vi "[Bug] Double FFT Mesurament RT with Frequency Linearization & BackNoise Remove Test.vi"() -> ()   [LabVIEW 2014]
uses:
  <vilib>/Platform/TimedLoop/XDataNode/timing_clust.ctl
  <vilib>/Platform/TimedLoop/XDataNode/nitl_modes.ctl
  <vilib>/Platform/TimedLoop/XDataNode/wakeup.ctl
  <vilib>/FPGAPlugInAG/sbRIO-9636/niLvFpga_Open_sbRIO-9636.vi
  <vilib>/rvi/interface/common/dynamic/niFpgaDynamicAddResources.vi
  <vilib>/FPGAPlugInAG/Dynamic/niLvFpga_Reset_Dynamic.vi
  <vilib>/Utility/error.llb/Error Cluster From Error Code.vi
  <vilib>/rvi/errors/niLvFpgaAdjustHostInterfaceError.vi
  <vilib>/rvi/interface/common/niFpgaWaitOnOcc.vi
  <vilib>/FPGAPlugInAG/Dynamic/niLvFpga_Run_Dynamic.vi
  <vilib>/FPGAPlugInAG/Dynamic/niLvFpga_Abort_Dynamic.vi
  <vilib>/FPGAPlugInAG/Dynamic/niLvFpga_Close_Dynamic.vi
  <vilib>/rvi/interface/nirviOpenFPGA/nirviOpenFPGA.xnode
  FPGA Bitfiles/LaserDistanceSen_FPGATarget_DoubleFFTMesuram_6dDziXQAIGE.lvbitx
  FPGA Target/Test VIs/Double FFT Mesurament Test with Background Noise Remove.vi
  <vilib>/rvi/interface/nirviMethod/nirviMethod.xnode
  <vilib>/rvi/interface/nirviReadWriteControl/nirviReadWriteControl.xnode
  <vilib>/Platform/TimedLoop/XDataNode/XDataNode.xnode
  <vilib>/rvi/interface/nirviCloseFPGA/nirviCloseFPGA.xnode
  <vilib>/FPGAPlugInAG/Dynamic/niLvFpga_ConfigureFifo_Dynamic.vi
  <vilib>/rvi/errors/niLvFpgaMergeErrorWithErrorCode.vi
  <vilib>/FPGAPlugInAG/Dynamic/niLvFpga_StartFifo_Dynamic.vi
  <vilib>/rvi/interface/Simulation/niFpgaSimulationCallBeginRW.vi
  <vilib>/FPGAPlugInAG/Dynamic/niLvFpga_ReadFifo_Dynamic.vi
  <vilib>/Platform/TimedLoop/XDataNode/XDNodeRunTimeDep.lvlib
  NiFpgaLv.dll
panel:
  in  "polynomial order":i32=3
  in  "side points":i32=6
  out "2^(n-bit) misure mediate":dbl
  in  "n-bit":i32=10
  in  "SubtractionType":T1(ring)
  out "Fondo Signal":dbl[](graph)
  in  "LowPass Filter: Low cutoff frequency":dbl=20000.0 format="%#_13g"
  in  "PolyFitting: Poly Grade":dbl=12.0
  in  "Scale Factor Rising":dbl=0.5
  out "2) Std Dev":dbl
  out "1) Std Dev":dbl
  in  "Scale Factor Falling":dbl=0.5
  in  "Triangolo dritto":bool=TRUE
  in  "Acrive  Smooth":bool
  out "Complete SkewTri":dbl[](graph)
  out "2) Tri edge RISING":dbl[](graph)
  out "1) Tri edge FALLING":dbl[](graph)
  out "1) Ext Mean Time Curve":dbl[](graph)
  out "2) Ext Mean Time Curve":dbl[](graph)
  out "2) Mean Freq Curve Rising":dbl[](graph)
  out "1) Mean Freq Curve Falling":dbl[](graph)
  out "2) Freq curve":dbl[](graph)
  out "1) Freq curve":dbl[](graph)
  in  "FFT Sliding Win Size":i32=128
  out "1) SmoothSubSig":dbl[](graph)
  out "2) SmoothSubSig":dbl[](graph)
  in  "Acrive Fit":bool=TRUE
  in  "Poly Order":i32=3
  in  "Side points":i32=13
  in  "Poly Grade":dbl=5.0
  out "2) Signal&Fit 2":dbl[][](graph)
  out "1) Signal&Fit":dbl[][](graph)
  in  "tieni premuto per":i32=1
  out "Current Sig lin":i32
  in  "Acrive Linearization":bool
  in  "# Measurements for Linearization":i32=10
  in  "?":bool
  out "maxbin_secondFFT":i32
  out "maxbin_firstFFT":i32
  out "f_rise":dbl
  out "f_fall":dbl
  out "f_mean":dbl
  out "Velocity (m/s)":dbl
  out "Distance (m)":dbl
  in  "Initial Latency points":u32(slide) scale=0.0..1249.0
  out "Second FFT (bin)":dbl[](graph)
  out "Second Signal (points) - Rising Triangular":dbl[](graph)
  out "First FFT (bin)":dbl[](graph)
  out "First Signal (points) - Falling Triangular":dbl[](graph)
  in  "Snapshot":bool
  in  "Windowing":T2(ring)
  in  "first bin":i32=5
  in  "last bin":i32=255
  in  "lower limit 2":u32(slide)=738 scale=625.0..738.0
  in  "lower limit 1":u32(slide)=113 scale=0.0..113.0
  # "-> TODO: Sistemare problema della finestra di acquisizione ritardata"
  # "Estrazione del rumore di fondo (Background noise extraction)"
  # "Sav Golay Filter"
  # "WARNING:\nOnce pressed wait untill the end of operation"
  # "OFFLINE parameters"
  # "Triangolo storto\nda costante"
  # "Max Detection FFT bin range"
  # "ONLINE parameters"
  # "Se la sottrazione del fondo non è eseguita su FPGA.\n Attivarla per eseguirla lato RT"
  # "Smoothing (S-G Params)"
  # "Fitting"
  # "ONLY POWER OF 2"
  # "Min: 2 Max: 256 (2, 4, 8, 16, 32, 64, 128, 256)"
  # "LINEARIZATION FINAL RESULTS"
  # "dev standard (max-min)"
  # "%"
  # "%"
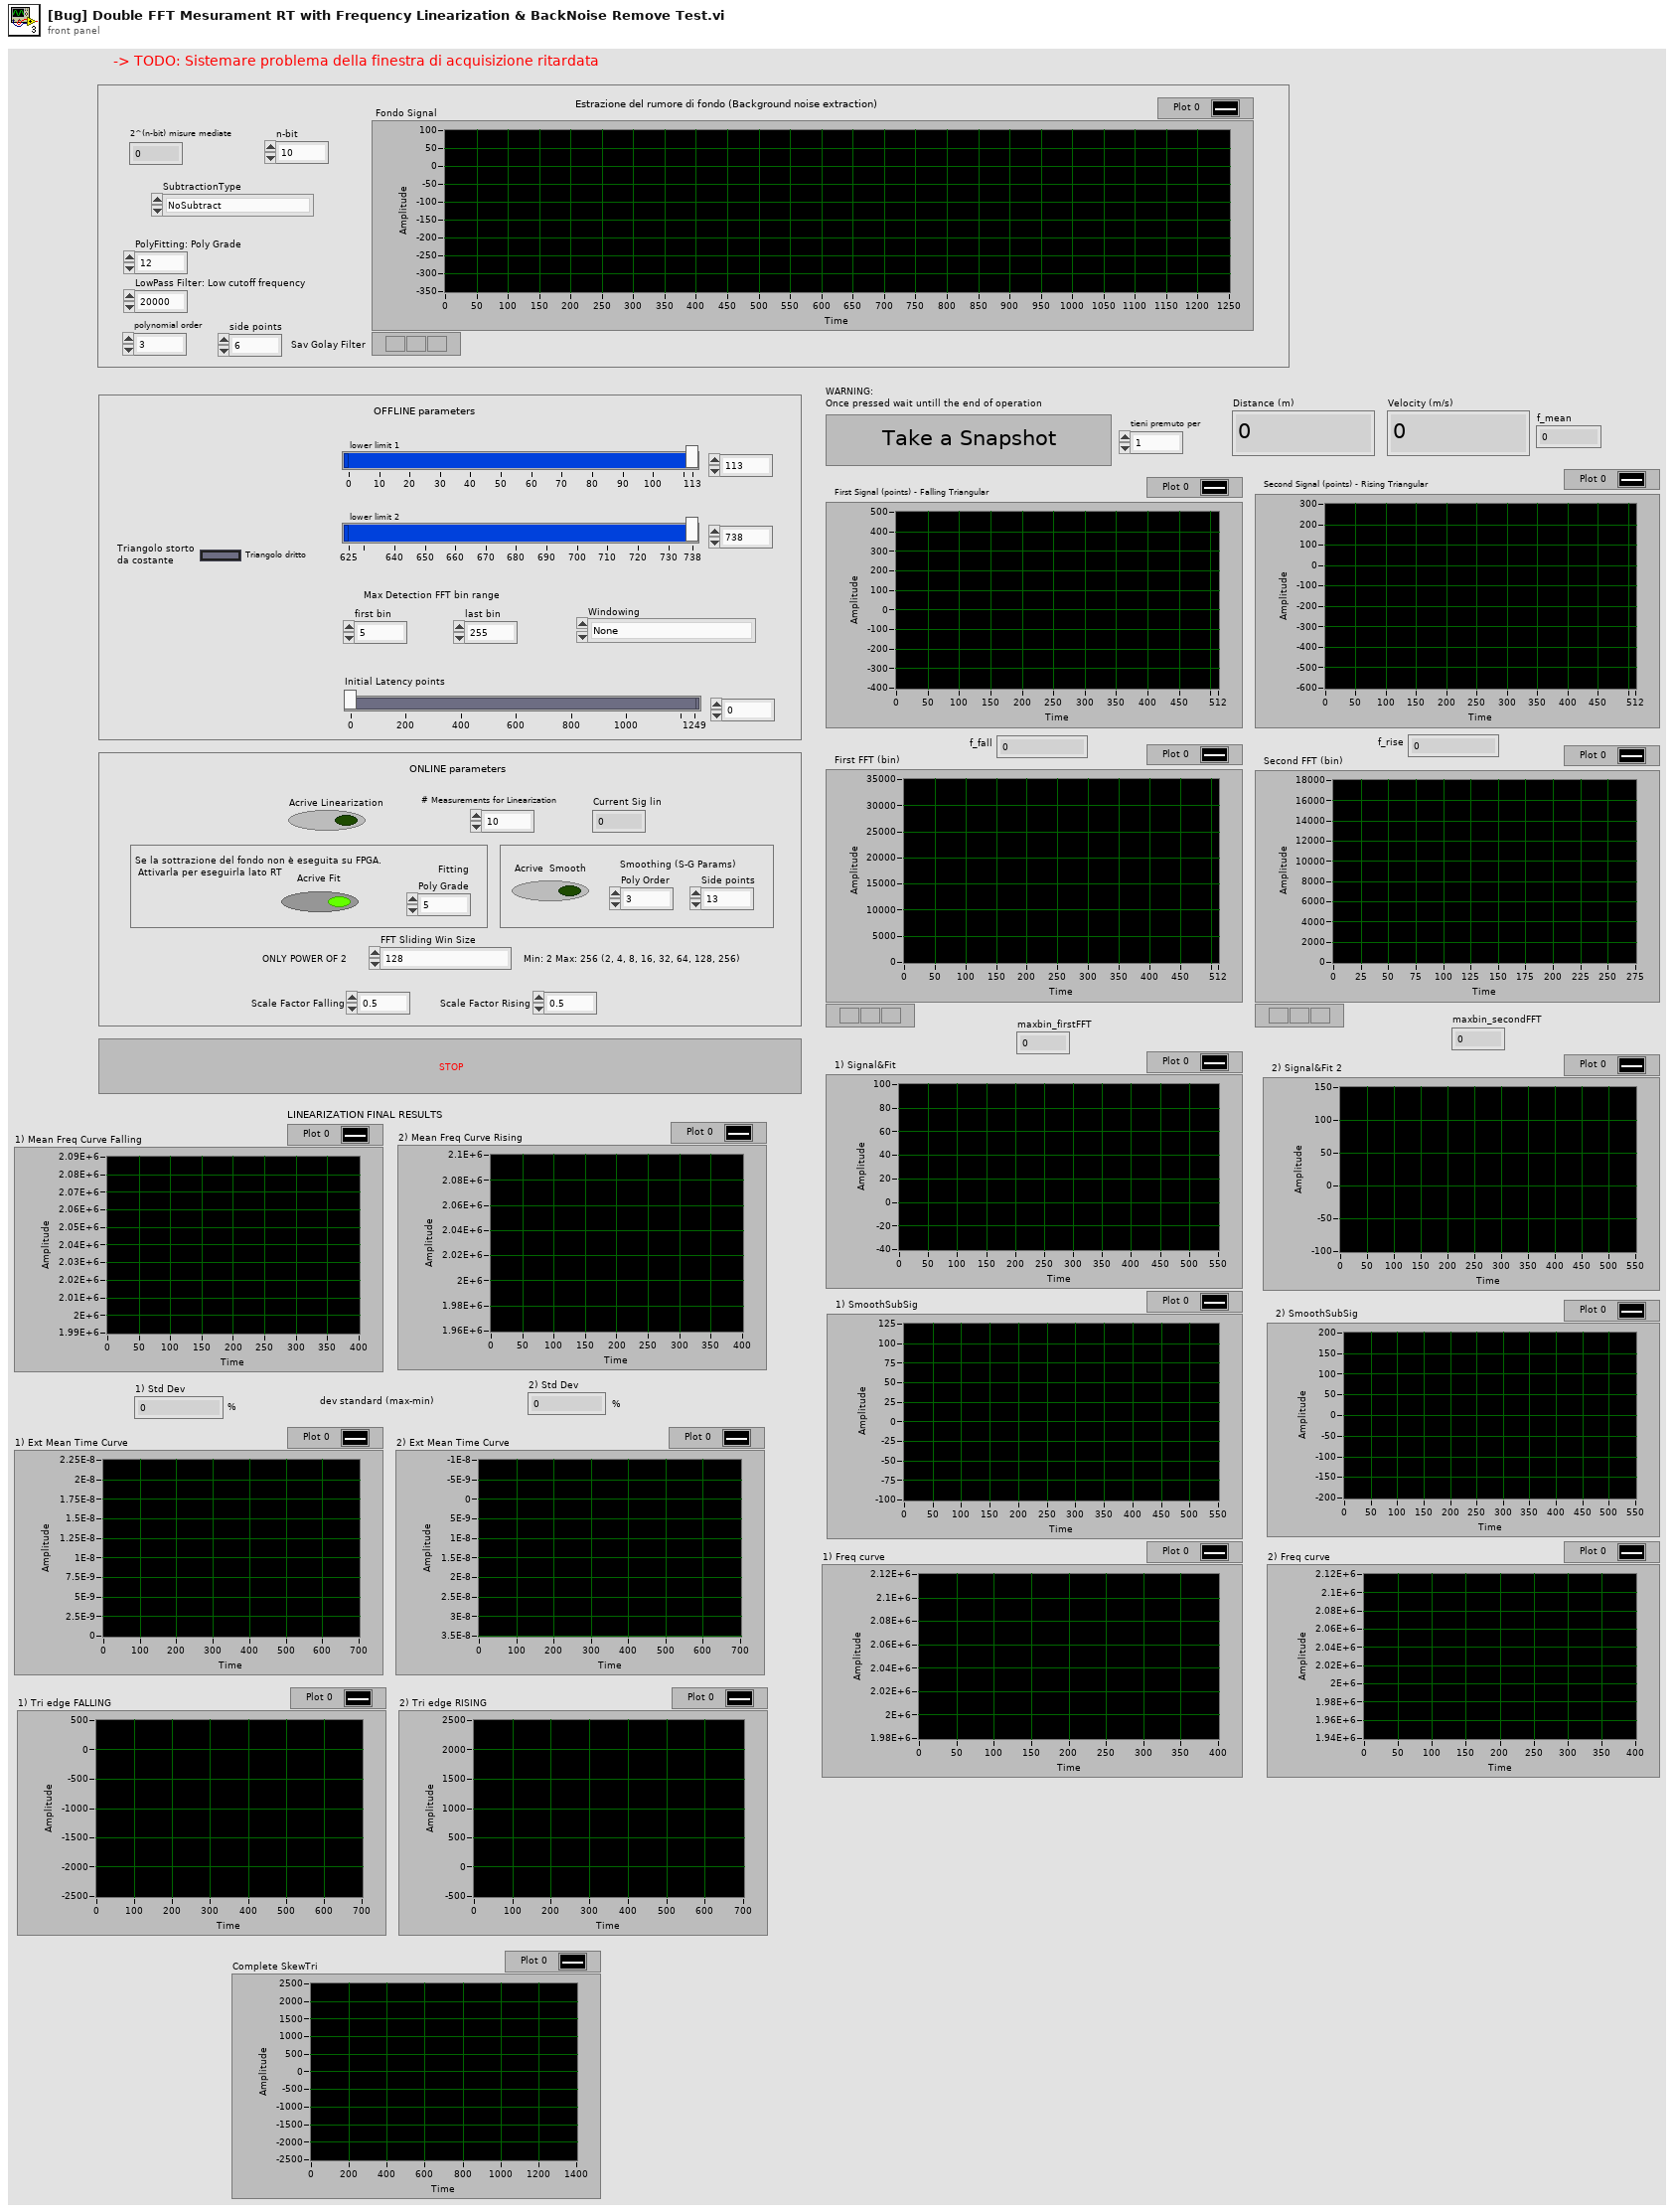
[diagram p1: front panel]
types:
  T1 = enum16{"NoSubtract", "StartingCurve", "LowPass", "PolyFitting", "SavGolay"}
  T2 = enum16{"None", "Hanning", "Hamming", "Blackman", "Blackman-Harris"}
  T3 = typedef "XDNodeRunTimeDep.lvlib/timing_clust.ctl" = cluster{"Expected End [f-1]":u64, "Actual End [f-1]":u64, "Finished Late? [f-1]":bool, "Expected End [i-1]":u64, "Actual End [i-1]":u64, "Finished Late? [i-1]":bool, "Expected Start [i]":u64, "Actual Start [i]":u64, "Expected Start [f]":u64, "Actual Start [f]":u64, "Source Name":string, "Structure Name":string, "Period":i64, "Deadline":i64, "Offset":i64, "Start":i64, "Priority":i32, "Timeout":i32, "Mode":T4, "Wakeup Reason":T5, "Error":errorcluster, "Source Type":string, "Secondary Source Type":string, "Global End Time":u64, "Global Start Time":u64, "Frame Duration":u64, "Iteration Duration":u64, "Assigned CPU":i32, "I/O Scan Engine Mode":u32}
  T4 = typedef "XDNodeRunTimeDep.lvlib/nitl_modes.ctl" = enum32{"No Change", "Process missed periods, maintain original phase", "Discard missed periods, maintain original phase", "Process missed periods, ignore original phase", "Discard missed periods, ignore original phase"}
  T5 = typedef "XDNodeRunTimeDep.lvlib/wakeup.ctl" = enum32{"Normal", "Aborted", "Asynchronous wakeup", "Timing source error", "Timed loop error", "Timeout"}
  T6 = typedef "NI_Matrix.lvlib/RealMatrix.ctl" = dbl[][]
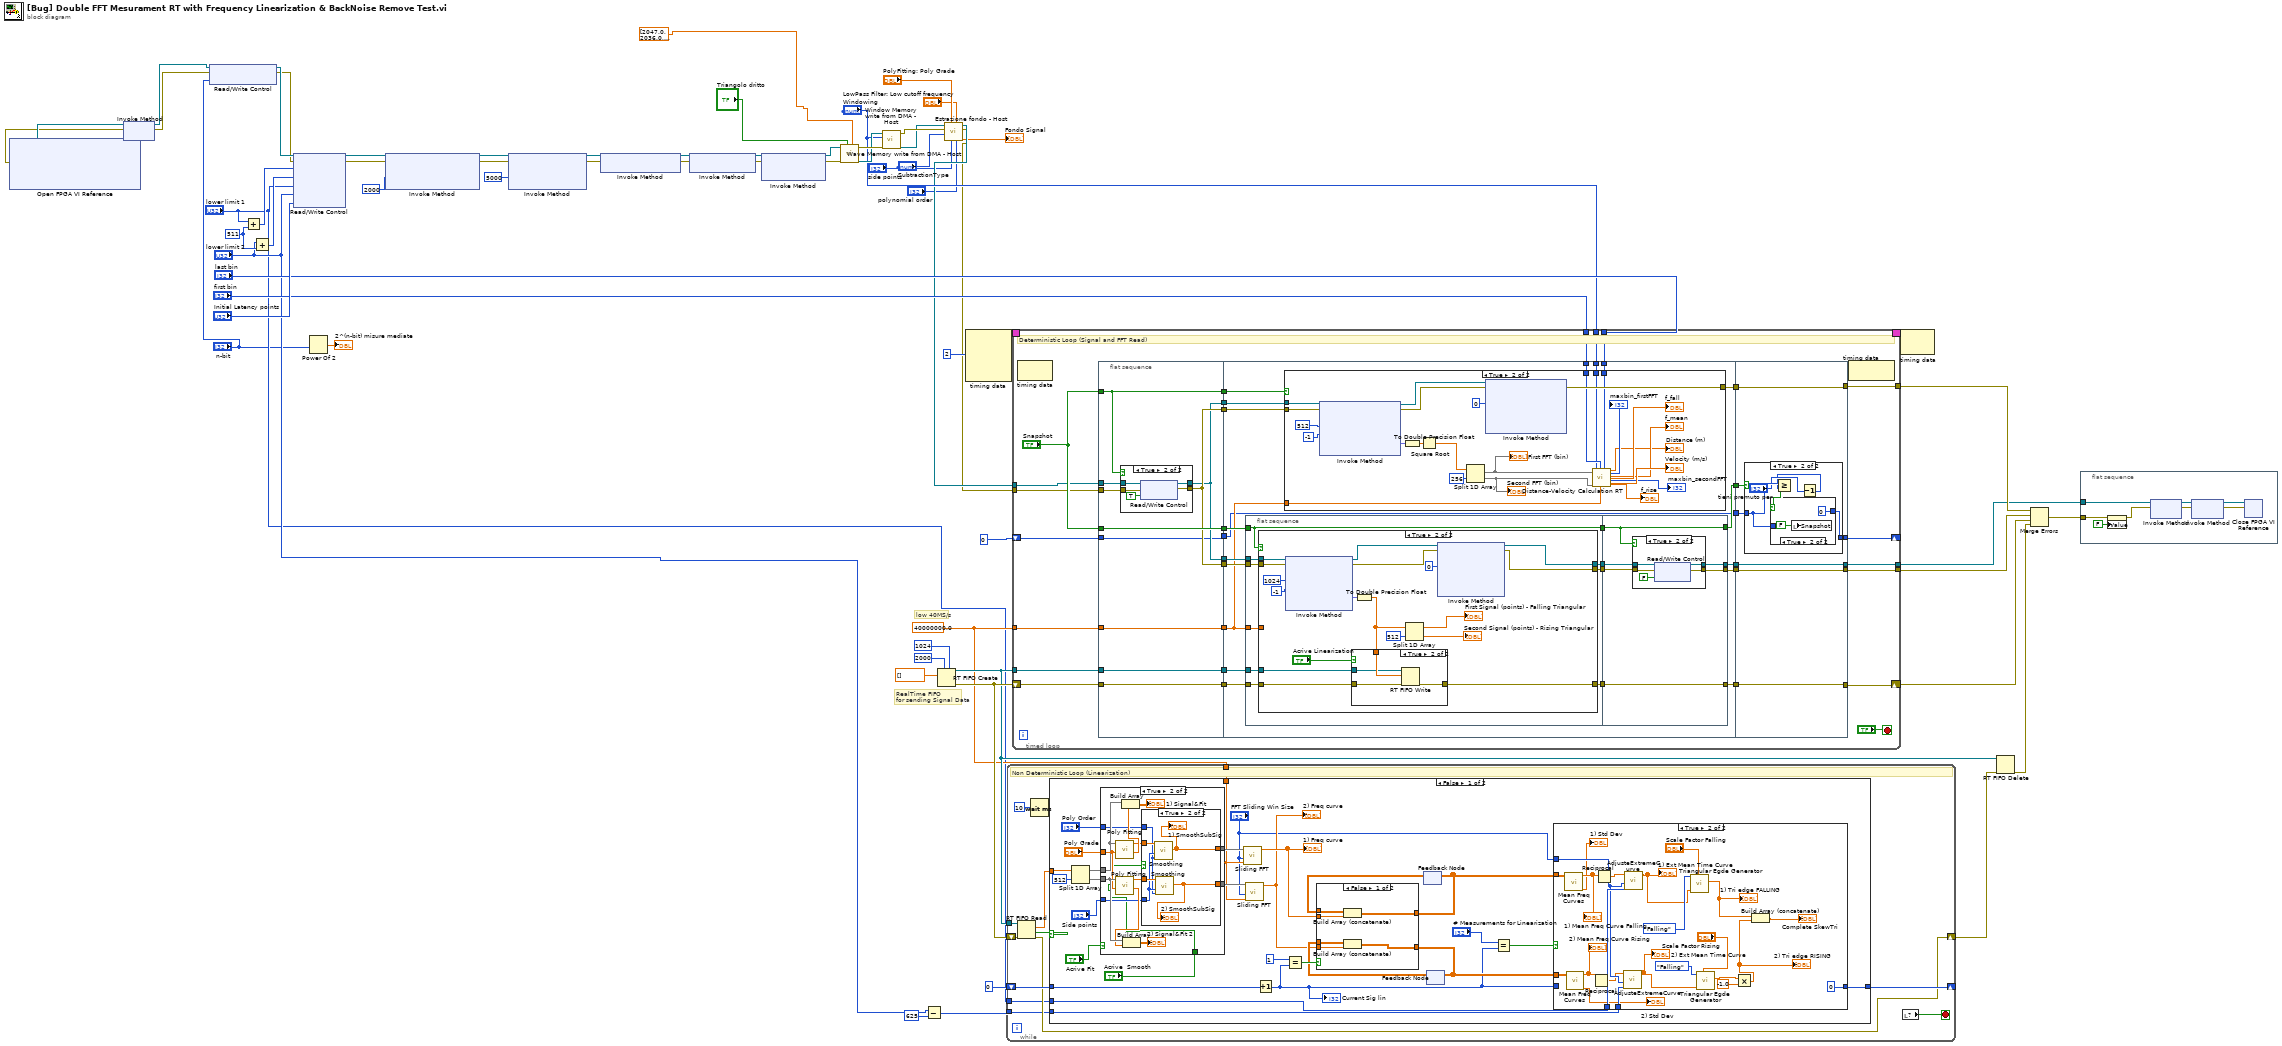
[diagram p0: block diagram]
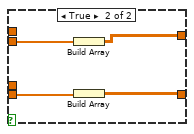
[diagram p5: hidden frame]
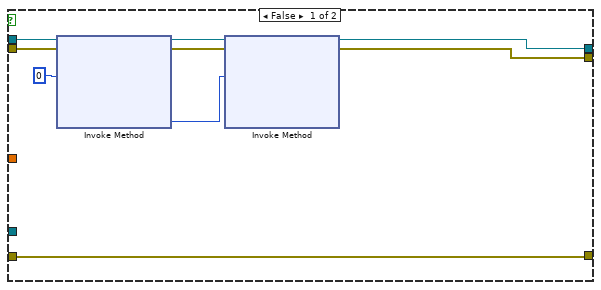
[diagram p8: hidden frame]
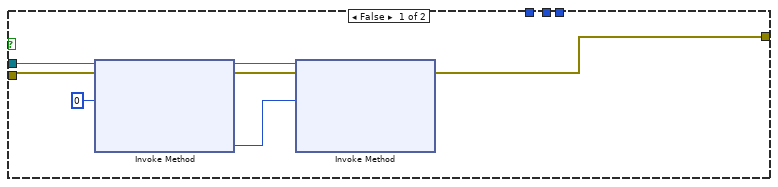
[diagram p11: hidden frame]
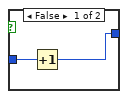
[diagram p13: hidden frame]
diagram:
  w63 = u32 511 ("y")
  w22 = 40000000.0 ("Sample Rate (S/s)")
  # "RealTime FIFO \nfor sending Signal Data"
  # "low 40MS/s"
  n1 = xnode "Open FPGA VI Reference"() -> ("FPGA VI Reference Out"=w7:refnum<k20>, "error out"=w6:errorcluster)  [unwired: 2 in]
  n2 = xnode "Invoke Method"("FPGA VI Reference In"=w7, "error in"=w6) -> ("FPGA VI Reference Out"=w4:refnum<k20>, "error out"=w2:errorcluster)
  n3 = xnode "Read/Write Control"("FPGA VI Reference In"=w4, "error in"=w2, "n-bit (2^nbit medie)"="n-bit") -> ("FPGA VI Reference Out"=w3:refnum<k20>, "error out"=w1:errorcluster)
  n4 = Add(x="lower limit 1", y=w63) -> (x+y=w65:u32)
  n5 = Add(x="lower limit 2", y=w63) -> (x+y=w64:u32)
  n6 = xnode "Read/Write Control"("FPGA VI Reference In"=w3, "error in"=w1, "upper limit 1"=w65, "upper limit 2"=w64, "lower limit 1"="lower limit 1", "lower limit 2"="lower limit 2", "Latency points"="Initial Latency points") -> ("FPGA VI Reference Out"=w62:refnum<k20>, "error out"=w61:errorcluster)
  n7 = Power Of 2(x="n-bit") -> (2^x=→"2^(n-bit) misure mediate":dbl)
  n8 = xnode "Invoke Method"("FPGA VI Reference In"=w62, "error in"=w61, "Requested Depth"=u32 2000) -> ("FPGA VI Reference Out"=w40:refnum<k20>, "error out"=w41:errorcluster)  [unwired: 1 out]
  n9 = xnode "Invoke Method"("FPGA VI Reference In"=w40, "error in"=w41, "Requested Depth"=u32 5000) -> ("FPGA VI Reference Out"=w54:refnum<k20>, "error out"=w55:errorcluster)  [unwired: 1 out]
  n10 = xnode "Invoke Method"("FPGA VI Reference In"=w54, "error in"=w55) -> ("FPGA VI Reference Out"=w38:refnum<k20>, "error out"=w39:errorcluster)
  n11 = xnode "Invoke Method"("FPGA VI Reference In"=w38, "error in"=w39) -> ("FPGA VI Reference Out"=w52:refnum<k20>, "error out"=w53:errorcluster)
  n12 = xnode "Invoke Method"("FPGA VI Reference In"=w52, "error in"=w53) -> ("FPGA VI Reference Out"=w58:refnum<k20>, "error out"=w57:errorcluster)  [unwired: 1 in]
  n13 = call "Wave Memory write from DMA - Host.vi"("Custom Triangular Signal (fal-ris)"=dbl[] [2047.0, 2036.0, 2024.0, 2013.0, 2002.0, 1990.0, 1979.0, 1968.0, 1956.0, 1945.0, 1934.0, 1923.0, 1912.0, 1900.0, 1889.0, 1878.0, 1867.0, 1856.0, 1845.0, 1833.0, 1822.0, 1811.0, 1800.0, 1789.0, 1778.0, 1767.0, 1756.0, 1745.0, 1734.0, 1723.0, 1712.0, 1702.0, 1691.0, 1680.0, 1669.0, 1658.0, 1647.0, 1636.0, 1626.0, 1615.0, 1604.0, 1593.0, 1583.0, 1572.0, 1561.0, 1550.0, 1540.0, 1529.0, 1518.0, 1508.0, 1497.0, 1487.0, 1476.0, 1465.0, 1455.0, 1444.0, 1434.0, 1423.0, 1413.0, 1402.0, 1392.0, 1381.0, 1371.0, 1360.0, 1350.0, 1340.0, 1329.0, 1319.0, 1309.0, 1298.0, 1288.0, 1278.0, 1267.0, 1257.0, 1247.0, 1237.0, 1226.0, 1216.0, 1206.0, 1196.0, 1186.0, 1176.0, 1165.0, 1155.0, 1145.0, 1135.0, 1125.0, 1115.0, 1105.0, 1095.0, 1085.0, 1075.0, 1065.0, 1055.0, 1045.0, 1035.0, 1025.0, 1015.0, 1006.0, 996.0, 986.0, 976.0, 966.0, 956.0, 947.0, 937.0, 927.0, 917.0, 908.0, 898.0, 888.0, 879.0, 869.0, 859.0, 850.0, 837.0, 826.0, 816.0, 804.0, 796.0, 788.0, 778.0, 769.0, 758.0, 750.0, 743.0, 733.0, 724.0, 717.0, 709.0, 701.0, 693.0, 686.0, 677.0, 669.0, 661.0, 653.0, 645.0, 638.0, 630.0, 622.0, 615.0, 607.0, 599.0, 592.0, 583.0, 576.0, 569.0, 561.0, 554.0, 547.0, 539.0, 532.0, 525.0, 518.0, 509.0, 501.0, 492.0, 486.0, 478.0, 471.0, 463.0, 456.0, 450.0, 442.0, 435.0, 429.0, 421.0, 415.0, 408.0, 401.0, 394.0, 388.0, 381.0, 375.0, 368.0, 361.0, 355.0, 349.0, 342.0, 336.0, 330.0, 323.0, 317.0, 311.0, 304.0, 298.0, 292.0, 286.0, 279.0, 273.0, 267.0, 261.0, 255.0, 249.0, 242.0, 236.0, 230.0, 224.0, 218.0, 212.0, 206.0, 200.0, 194.0, 187.0, 181.0, 175.0, 169.0, 163.0, 157.0, 150.0, 144.0, 138.0, 132.0, 125.0, 119.0, 113.0, 107.0, 101.0, 95.0, 88.0, 82.0, 77.0, 71.0, 65.0, 59.0, 53.0, 47.0, 41.0, 35.0, 29.0, 23.0, 18.0, 11.0, 6.0, 0.0, -6.0, -12.0, -18.0, -23.0, -29.0, -35.0, -41.0, -47.0, -52.0, -58.0, -64.0, -69.0, -75.0, -81.0, -87.0, -92.0, -98.0, -104.0, -109.0, -115.0, -121.0, -126.0, -132.0, -138.0, -144.0, -149.0, -155.0, -161.0, -166.0, -172.0, -177.0, -183.0, -189.0, -194.0, -200.0, -205.0, -211.0, -216.0, -222.0, -227.0, -233.0, -238.0, -244.0, -249.0, -255.0, -260.0, -266.0, -271.0, -277.0, -283.0, -288.0, -294.0, -299.0, -304.0, -310.0, -315.0, -321.0, -326.0, -331.0, -337.0, -342.0, -348.0, -353.0, -358.0, -364.0, -369.0, -375.0, -380.0, -385.0, -391.0, -396.0, -402.0, -407.0, -413.0, -418.0, -423.0, -429.0, -434.0, -439.0, -445.0, -450.0, -456.0, -461.0, -466.0, -472.0, -477.0, -483.0, -488.0, -493.0, -499.0, -504.0, -510.0, -515.0, -520.0, -526.0, -531.0, -537.0, -542.0, -548.0, -553.0, -558.0, -564.0, -569.0, -574.0, -580.0, -585.0, -590.0, -596.0, -601.0, -606.0, -612.0, -617.0, -622.0, -628.0, -633.0, -638.0, -644.0, -649.0, -654.0, -660.0, -665.0, -670.0, -676.0, -681.0, -686.0, -692.0, -697.0, -702.0, -708.0, -713.0, -718.0, -723.0, -729.0, -734.0, -739.0, -744.0, -750.0, -755.0, -760.0, -765.0, -771.0, -776.0, -781.0, -786.0, -792.0, -797.0, -802.0, -807.0, -812.0, -818.0, -823.0, -828.0, -833.0, -839.0, -844.0, -849.0, -854.0, -859.0, -865.0, -870.0, -875.0, -880.0, -885.0, -891.0, -896.0, -901.0, -906.0, -911.0, -916.0, -922.0, -927.0, -932.0, -937.0, -943.0, -948.0, -953.0, -958.0, -963.0, -969.0, -974.0, -979.0, -984.0, -989.0, -995.0, -1000.0, -1005.0, -1010.0, -1015.0, -1021.0, -1026.0, -1031.0, -1036.0, -1041.0, -1047.0, -1052.0, -1057.0, -1062.0, -1067.0, -1073.0, -1078.0, -1083.0, -1088.0, -1093.0, -1099.0, -1104.0, -1109.0, -1114.0, -1119.0, -1124.0, -1130.0, -1135.0, -1140.0, -1145.0, -1150.0, -1156.0, -1161.0, -1166.0, -1171.0, -1176.0, -1182.0, -1187.0, -1192.0, -1197.0, -1202.0, -1207.0, -1213.0, -1218.0, -1223.0, -1228.0, -1233.0, -1238.0, -1244.0, -1249.0, -1254.0, -1259.0, -1264.0, -1269.0, -1275.0, -1280.0, -1285.0, -1290.0, -1295.0, -1300.0, -1305.0, -1311.0, -1316.0, -1321.0, -1326.0, -1331.0, -1336.0, -1342.0, -1347.0, -1352.0, -1357.0, -1362.0, -1367.0, -1372.0, -1378.0, -1383.0, -1388.0, -1393.0, -1398.0, -1403.0, -1408.0, -1414.0, -1419.0, -1424.0, -1429.0, -1434.0, -1439.0, -1444.0, -1450.0, -1455.0, -1460.0, -1465.0, -1470.0, -1475.0, -1480.0, -1486.0, -1491.0, -1496.0, -1501.0, -1506.0, -1511.0, -1516.0, -1522.0, -1527.0, -1532.0, -1537.0, -1542.0, -1547.0, -1552.0, -1558.0, -1563.0, -1568.0, -1573.0, -1578.0, -1583.0, -1588.0, -1593.0, -1599.0, -1604.0, -1609.0, -1614.0, -1619.0, -1624.0, -1629.0, -1634.0, -1640.0, -1645.0, -1650.0, -1655.0, -1660.0, -1665.0, -1670.0, -1675.0, -1681.0, -1686.0, -1691.0, -1696.0, -1701.0, -1706.0, -1711.0, -1716.0, -1722.0, -1727.0, -1732.0, -1737.0, -1742.0, -1747.0, -1752.0, -1757.0, -1762.0, -1768.0, -1773.0, -1778.0, -1783.0, -1788.0, -1793.0, -1798.0, -1803.0, -1808.0, -1814.0, -1819.0, -1824.0, -1829.0, -1834.0, -1839.0, -1844.0, -1849.0, -1854.0, -1859.0, -1865.0, -1870.0, -1875.0, -1880.0, -1885.0, -1890.0, -1895.0, -1900.0, -1905.0, -1911.0, -1916.0, -1921.0, -1926.0, -1931.0, -1936.0, -1941.0, -1946.0, -1951.0, -1956.0, -1961.0, -1967.0, -1972.0, -1977.0, -1982.0, -1987.0, -1992.0, -1997.0, -2002.0, -2007.0, -2012.0, -2017.0, -2023.0, -2028.0, -2033.0, -2038.0, -2043.0, -2048.0, -2047.0, -2034.0, -2021.0, -2009.0, -1996.0, -1983.0, -1970.0, -1957.0, -1945.0, -1932.0, -1919.0, -1907.0, -1894.0, -1881.0, -1869.0, -1856.0, -1844.0, -1831.0, -1819.0, -1806.0, -1794.0, -1781.0, -1769.0, -1757.0, -1744.0, -1732.0, -1719.0, -1707.0, -1695.0, -1682.0, -1670.0, -1658.0, -1646.0, -1634.0, -1621.0, -1609.0, -1597.0, -1585.0, -1573.0, -1561.0, -1549.0, -1537.0, -1525.0, -1513.0, -1501.0, -1489.0, -1477.0, -1465.0, -1453.0, -1441.0, -1429.0, -1417.0, -1405.0, -1394.0, -1382.0, -1370.0, -1358.0, -1347.0, -1335.0, -1323.0, -1312.0, -1300.0, -1288.0, -1277.0, -1265.0, -1254.0, -1242.0, -1231.0, -1219.0, -1208.0, -1196.0, -1185.0, -1173.0, -1162.0, -1150.0, -1139.0, -1128.0, -1116.0, -1105.0, -1094.0, -1083.0, -1071.0, -1060.0, -1049.0, -1038.0, -1027.0, -1015.0, -1004.0, -993.0, -982.0, -971.0, -960.0, -949.0, -938.0, -927.0, -916.0, -905.0, -894.0, -883.0, -873.0, -862.0, -851.0, -840.0, -829.0, -819.0, -808.0, -797.0, -786.0, -776.0, -765.0, -754.0, -744.0, -733.0, -722.0, -712.0, -697.0, -685.0, -674.0, -661.0, -652.0, -643.0, -632.0, -622.0, -610.0, -602.0, -594.0, -583.0, -574.0, -566.0, -558.0, -550.0, -542.0, -534.0, -525.0, -516.0, -507.0, -499.0, -491.0, -483.0, -475.0, -467.0, -459.0, -451.0, -443.0, -435.0, -426.0, -419.0, -411.0, -404.0, -396.0, -388.0, -381.0, -373.0, -366.0, -359.0, -349.0, -341.0, -331.0, -325.0, -317.0, -309.0, -301.0, -295.0, -288.0, -280.0, -273.0, -266.0, -259.0, -252.0, -246.0, -239.0, -231.0, -225.0, -219.0, -212.0, -205.0, -199.0, -192.0, -186.0, -180.0, -173.0, -167.0, -161.0, -155.0, -148.0, -142.0, -136.0, -130.0, -124.0, -118.0, -112.0, -106.0, -100.0, -94.0, -88.0, -82.0, -76.0, -70.0, -64.0, -58.0, -52.0, -46.0, -40.0, -34.0, -28.0, -21.0, -15.0, -9.0, -3.0, 2.0, 9.0, 15.0, 21.0, 27.0, 33.0, 39.0, 45.0, 51.0, 57.0, 63.0, 69.0, 75.0, 81.0, 86.0, 92.0, 98.0, 103.0, 110.0, 116.0, 121.0, 127.0, 133.0, 138.0, 144.0, 149.0, 155.0, 161.0, 166.0, 172.0, 177.0, 183.0, 189.0, 194.0, 200.0, 205.0, 211.0, 216.0, 221.0, 227.0, 232.0, 238.0, 243.0, 249.0, 254.0, 259.0, 265.0, 270.0, 276.0, 281.0, 286.0, 292.0, 297.0, 303.0, 308.0, 314.0, 319.0, 324.0, 329.0, 335.0, 340.0, 345.0, 351.0, 356.0, 361.0, 366.0, 371.0, 377.0, 382.0, 387.0, 392.0, 397.0, 403.0, 408.0, 413.0, 418.0, 423.0, 429.0, 434.0, 439.0, 444.0, 449.0, 454.0, 459.0, 464.0, 469.0, 474.0, 479.0, 484.0, 489.0, 494.0, 499.0, 504.0, 509.0, 514.0, 520.0, 525.0, 530.0, 535.0, 540.0, 545.0, 550.0, 555.0, 560.0, 565.0, 570.0, 575.0, 580.0, 585.0, 590.0, 595.0, 600.0, 605.0, 610.0, 615.0, 620.0, 625.0, 630.0, 636.0, 641.0, 646.0, 651.0, 656.0, 661.0, 666.0, 671.0, 676.0, 681.0, 686.0, 691.0, 696.0, 701.0, 706.0, 711.0, 716.0, 721.0, 726.0, 731.0, 736.0, 741.0, 746.0, 751.0, 756.0, 761.0, 765.0, 770.0, 775.0, 780.0, 785.0, 790.0, 795.0, 800.0, 805.0, 810.0, 815.0, 820.0, 825.0, 829.0, 834.0, 839.0, 844.0, 849.0, 854.0, 859.0, 864.0, 868.0, 873.0, 878.0, 883.0, 888.0, 893.0, 897.0, 902.0, 907.0, 912.0, 917.0, 921.0, 926.0, 931.0, 936.0, 941.0, 945.0, 950.0, 955.0, 960.0, 965.0, 969.0, 974.0, 979.0, 984.0, 988.0, 993.0, 998.0, 1003.0, 1007.0, 1012.0, 1017.0, 1022.0, 1027.0, 1031.0, 1036.0, 1041.0, 1046.0, 1051.0, 1055.0, 1060.0, 1065.0, 1070.0, 1075.0, 1079.0, 1084.0, 1089.0, 1094.0, 1098.0, 1103.0, 1108.0, 1113.0, 1118.0, 1122.0, 1127.0, 1132.0, 1137.0, 1141.0, 1146.0, 1151.0, 1156.0, 1161.0, 1165.0, 1170.0, 1175.0, 1180.0, 1184.0, 1189.0, 1194.0, 1199.0, 1204.0, 1208.0, 1213.0, 1218.0, 1223.0, 1227.0, 1232.0, 1237.0, 1242.0, 1246.0, 1251.0, 1256.0, 1261.0, 1265.0, 1270.0, 1275.0, 1280.0, 1284.0, 1289.0, 1294.0, 1299.0, 1303.0, 1308.0, 1313.0, 1318.0, 1322.0, 1327.0, 1332.0, 1336.0, 1341.0, 1346.0, 1351.0, 1355.0, 1360.0, 1365.0, 1370.0, 1374.0, 1379.0, 1384.0, 1388.0, 1393.0, 1398.0, 1403.0, 1407.0, 1412.0, 1417.0, 1421.0, 1426.0, 1431.0, 1436.0, 1440.0, 1445.0, 1450.0, 1454.0, 1459.0, 1464.0, 1469.0, 1473.0, 1478.0, 1483.0, 1487.0, 1492.0, 1497.0, 1502.0, 1506.0, 1511.0, 1516.0, 1520.0, 1525.0, 1530.0, 1535.0, 1539.0, 1544.0, 1549.0, 1553.0, 1558.0, 1563.0, 1567.0, 1572.0, 1577.0, 1582.0, 1586.0, 1591.0, 1596.0, 1600.0, 1605.0, 1610.0, 1614.0, 1619.0, 1624.0, 1628.0, 1633.0, 1638.0, 1643.0, 1647.0, 1652.0, 1657.0, 1661.0, 1666.0, 1671.0, 1675.0, 1680.0, 1685.0, 1689.0, 1694.0, 1699.0, 1703.0, 1708.0, 1713.0, 1717.0, 1722.0, 1727.0, 1731.0, 1736.0, 1741.0, 1746.0, 1750.0, 1755.0, 1760.0, 1764.0, 1769.0, 1774.0, 1778.0, 1783.0, 1788.0, 1792.0, 1797.0, 1802.0, 1806.0, 1811.0, 1816.0, 1820.0, 1825.0, 1830.0, 1834.0, 1839.0, 1844.0, 1848.0, 1853.0, 1858.0, 1862.0, 1867.0, 1871.0, 1876.0, 1881.0, 1885.0, 1890.0, 1895.0, 1899.0, 1904.0, 1909.0, 1913.0, 1918.0, 1923.0, 1927.0, 1932.0, 1937.0, 1941.0, 1946.0, 1951.0, 1955.0, 1960.0, 1965.0, 1969.0, 1974.0, 1978.0, 1983.0, 1988.0, 1992.0, 1997.0, 2002.0, 2006.0, 2011.0, 2016.0, 2020.0, 2025.0, 2029.0, 2034.0, 2039.0, 2043.0, 2048.0] ("Complete SkewTri"), "Triangolo dritto?"="Triangolo dritto", "error in"=w57, "FPGA VI Reference In"=w58) -> ("FPGA VI Reference Out"=w43:refnum<k20>, "error out"=w56:errorcluster)  [unwired: 5 in, 1 out]
  n14 = call "Window Memory write from DMA - Host.vi"("error in"=w56, "Enum"="Windowing", "FPGA VI Reference In"=w43) -> ("FPGA VI Reference Out"=w17:refnum<k20>, "error out"=w18:errorcluster)  [unwired: 5 in, 2 out]
  n15 = Subtract(x="lower limit 2", y=u32 625) -> (x-y=w24:u32)
  n16 = RT FIFO Create(1:dbl[] [] ("double precision float"), 4:u32 2000 ("size (10)"), 6:u32 1024 ("elements in array (1)")) -> (8:w30:refnum<k33>, 11:w32:errorcluster)  [unwired: 5 in, 1 out]
  n17 = call "Estrazione fondo - Host.vi"("polynomial order"="polynomial order", "LowPass Filter: Low cutoff frequency"="LowPass Filter: Low cutoff frequency", "side points"="side points", "PolyFitting: Poly Grade"="PolyFitting: Poly Grade", "SubtractionType"="SubtractionType", "error in"=w18, "FPGA VI Reference In"=w17) -> ("Fondo Signal"=→"Fondo Signal":dbl[], "error out"=w15:errorcluster, "FPGA VI Reference Out"=w16:refnum<k20>)  [unwired: 1 in, 1 out]
  n18 = node-c288(i64 2 ("Period")) -> (w51:T3)  [unwired: 3 in]
  n19 = while {
    shift-right: [w69] -> w29
    shift-left: w32 -> [w71]
    tunnel: w30 -> [w76]
    shift-right: [w70] -> _
    shift-left: 0 -> [w74]
    tunnel: "lower limit 1" -> [w66]
    tunnel: w24 -> [w67]
    tunnel: w22 -> [w68]
    stop <- w75 stop-if-true
    # "Non Deterministic Loop (Linearization)"
    n20 = RT FIFO Read(0:w76, 3:w71) -> (9:w73:dbl[], 10:w72:bool, 11:w69:errorcluster)  [unwired: 2 in, 2 out]
    n21 = Wait (ms)(milliseconds to wait=u32 10 ("millisecond multiple")) -> ()  [unwired: 1 out]
    n22 = case shown="False" w72 {
      tunnel: w74 -> [w105 w164]
      tunnel: [w94 w164] -> w70
      tunnel: w73 -> [w103 _]
      tunnel: w68 -> [w84 _]
      tunnel: w67 -> [w81 _]
      tunnel: w66 -> [w80 _]
      frame False {
        n23 = Split 1D Array(array=w103, index=512) -> (first subarray=w92:dbl[], second subarray=w91:dbl[])
        n24 = case shown="True" "Acrive Fit" {
          tunnel: w92 -> [w107 w121]
          tunnel: w91 -> [w106 w117]
          tunnel: "Poly Grade" -> [_ w113]
          tunnel: "Side points" -> [_ w112]
          tunnel: "Poly Order" -> [_ w111]
          tunnel: [w106 w110] -> w85
          tunnel: [w107 w108] -> w86
          tunnel: "Acrive  Smooth" -> [_ w109]
          frame False {
          }
          frame True {
            n25 = call "Poly Fitting.vi"("Poly Grade"=w113, "Signal"=w121) -> ("Poly Signal"=w120:dbl[], "SubtractedSignal"=w115:dbl[])  [unwired: 8 in]
            n26 = call "Poly Fitting.vi"("Poly Grade"=w113, "Signal"=w117) -> ("Poly Signal"=w116:dbl[], "SubtractedSignal"=w114:dbl[])  [unwired: 8 in]
            n27 = Build Array(w121, w120) -> (→"1) Signal&Fit":dbl[][])
            n28 = Build Array(w117, w116) -> (→"2) Signal&Fit 2":dbl[][])
            n29 = case shown="True" w109 {
              tunnel: w115 -> [w123 w129]
              tunnel: w114 -> [w122 w128]
              tunnel: w112 -> [_ w127]
              tunnel: w111 -> [_ w126]
              tunnel: [w122 w125] -> w110
              tunnel: [w123 w124] -> w108
              frame False {
              }
              frame True {
                n30 = call "Smoothing.vi"("polynomial order"=w126, "side points"=w127, "SubtractedSignal"=w129) -> ("SubSmoothSignal"=w124:dbl[])  [unwired: 8 in]
                "1) SmoothSubSig" <- w124
                n31 = call "Smoothing.vi"("polynomial order"=w126, "side points"=w127, "SubtractedSignal"=w128) -> ("SubSmoothSignal"=w125:dbl[])  [unwired: 8 in]
                "2) SmoothSubSig" <- w125
              }
            }
          }
        }
        n32 = call "Sliding FFT.vi"("Sample Freq"=w84, "FFT Win Size"="FFT Sliding Win Size", "SubSmoothSignal"=w86) -> ("Freq samples"=w83:dbl[])  [unwired: 7 in, 1 out]
        "1) Freq curve" <- w83
        n33 = call "Sliding FFT.vi"("Sample Freq"=w84, "FFT Win Size"="FFT Sliding Win Size", "SubSmoothSignal"=w85) -> ("Freq samples"=w82:dbl[])  [unwired: 7 in, 1 out]
        "2) Freq curve" <- w82
        n34 = Increment(x=w105) -> (x+1=w95:i32)
        "Current Sig lin" <- w95
        n35 = Equal?(x=1, y=w95) -> (x = y?=w101:bool)
        n36 = feedback #1() -> (w100:T6)  [unwired: 1 in]
        n37 = feedback #2() -> (w99:T6)  [unwired: 1 in]
        n38 = case shown="False" w101 {
          tunnel: w82 -> [w158 w161]
          tunnel: w83 -> [w159 w163]
          tunnel: [w157 w160] -> w96
          tunnel: [w156 w162] -> w97
          tunnel: w100 -> [w155 _]
          tunnel: w99 -> [w154 _]
          frame False {
            n39 = Build Array (concatenate)(w155, w159) -> (w156:T6)
            n40 = Build Array (concatenate)(w154, w158) -> (w157:T6)
          }
          frame True {
            n41 = Build Array(w163) -> (w162:T6)
            n42 = Build Array(w161) -> (w160:T6)
          }
        }
        n43 = feedback-in #1(w97) -> ()
        n44 = feedback-in #2(w96) -> ()
        n45 = Equal?(x="# Measurements for Linearization", y=w95) -> (x = y?=w93:bool)
        n46 = case shown="True" w93 {
          tunnel: w97 -> [_ w132]
          tunnel: w96 -> [_ w131]
          tunnel: w95 -> [w130 _]
          tunnel: [w130 0] -> w94
          tunnel: w81 -> [_ w148]
          tunnel: w80 -> [_ w147]
          tunnel: "FFT Sliding Win Size" -> [_ w146]
          frame False {
          }
          frame True {
            n47 = call "Mean Freq Curves.vi"("Set of Freq samples"=w132) -> ("StdDev%"=→"1) Std Dev":dbl, "Mean Freq Curve"=w141:dbl[])  [unwired: 9 in]
            "1) Mean Freq Curve Falling" <- w141
            n48 = call "Mean Freq Curves.vi"("Set of Freq samples"=w131) -> ("StdDev%"=→"2) Std Dev":dbl, "Mean Freq Curve"=w143:dbl[])  [unwired: 9 in]
            "2) Mean Freq Curve Rising" <- w143
            n49 = Reciprocal(x=w143) -> (1/x=w142:dbl[])
            n50 = Reciprocal(x=w141) -> (1/x=w140:dbl[])
            n51 = call "AdjusteExtremeCurve.vi"("Init Bins Discarded"=w148, "FFT Size Window"=w146, "Freq sample"=w142) -> ("Extended Freq Sample"=w144:dbl[])  [unwired: 8 in]
            "2) Ext Mean Time Curve" <- w144
            n52 = call "AdjusteExtremeCurve.vi"("Init Bins Discarded"=w147, "FFT Size Window"=w146, "Freq sample"=w140) -> ("Extended Freq Sample"=w145:dbl[])  [unwired: 8 in]
            "1) Ext Mean Time Curve" <- w145
            n53 = call "Triangular Egde Generator.vi"("fattore"="Scale Factor Falling", "Sample values"=w145, "Triangular edge"=enum16{"Rising", "Falling"}."Falling") -> ("Skew Triangular"=w150:dbl[])  [unwired: 8 in]
            "1) Tri edge FALLING" <- w150
            n54 = call "Triangular Egde Generator.vi"("fattore"="Scale Factor Rising", "Sample values"=w144, "Triangular edge"=enum16{"Rising", "Falling"}."Falling") -> ("Skew Triangular"=w138:dbl[])  [unwired: 8 in]
            n55 = Multiply(x=w138, y=-1.0) -> (x*y=w137:dbl[])
            "2) Tri edge RISING" <- w137
            n56 = Build Array (concatenate)(w150, w137) -> (→"Complete SkewTri":dbl[])
          }
        }
      }
      frame True {
      }
    }
    n57 = local read item#18() -> (w75:bool)
  }
  n58 = timed-loop {
    tunnel: w16 -> [w191]
    tunnel: w15 -> [w192]
    tunnel: [w194] -> w48
    tunnel: w22 -> [w196]
    tunnel: [w195] -> w47
    timing: w51 -> [_]
    timing-out: [_] -> w50
    tunnel: "first bin" -> [w180]
    tunnel: "last bin" -> [w179]
    tunnel: [w177] -> w42
    tunnel: "Windowing" -> [w175]
    shift-right: [w169] -> w33
    shift-left: w32 -> [w171]
    tunnel: w30 -> [w173]
    shift-right: [w165] -> _
    shift-left: 0 -> [w167]
    stop <- "?" stop-if-true
    # "Deterministic Loop (Signal and FFT Read)"
    n59 = node-c288() -> ()  [unwired: 1 in, 1 out]
    n60 = flat-sequence {
      tunnel: w191 -> [w204]
      tunnel: w192 -> [w205]
      tunnel: "Snapshot" -> [w202]
      tunnel: "Snapshot" -> [w207]
      tunnel: w196 -> [w208]
      tunnel: [w206] -> w190
      tunnel: [w208] -> w189
      tunnel: [w207] -> w188
      tunnel: [w202] -> w187
      tunnel: [w206] -> w186
      tunnel: [w203] -> w185
      tunnel: [w203] -> w184
      tunnel: [w201] -> w174
      tunnel: w173 -> [w201]
      tunnel: [w200] -> w172
      tunnel: w171 -> [w200]
      tunnel: [w199] -> w168
      tunnel: w167 -> [w199]
      tunnel: w190 -> [w233]
      tunnel: w189 -> [w221]
      tunnel: w188 -> [w227]
      tunnel: w187 -> [w230]
      tunnel: w186 -> [w229]
      tunnel: w185 -> [w228]
      tunnel: w184 -> [w234]
      tunnel: [w232] -> w183
      tunnel: [w231] -> w182
      tunnel: [w226] -> w181
      tunnel: w180 -> [w225]
      tunnel: w179 -> [w224]
      tunnel: [w223] -> w176
      tunnel: w175 -> [w222]
      tunnel: w174 -> [w220]
      tunnel: w172 -> [w219]
      tunnel: [w217] -> w170
      tunnel: w168 -> [w216]
      tunnel: [w216] -> w166
      tunnel: [w329] -> w194
      tunnel: [w330] -> w195
      tunnel: w183 -> [w330]
      tunnel: w182 -> [w329]
      tunnel: w181 -> [w328]
      tunnel: [w327] -> w177
      tunnel: w176 -> [w327]
      tunnel: [w326] -> w169
      tunnel: w170 -> [w326]
      tunnel: w166 -> [w325]
      tunnel: [w324] -> w165
      frame #0 {
        n61 = case shown="True" w202 {
          tunnel: [w209 w214] -> w206
          tunnel: w205 -> [w209 w213]
          tunnel: w204 -> [w210 w212]
          tunnel: [w210 w211] -> w203
          frame False {
          }
          frame True {
            n62 = xnode "Read/Write Control"("FPGA VI Reference In"=w212, "error in"=w213, "snapshot"=TRUE) -> ("FPGA VI Reference Out"=w211:refnum<k20>, "error out"=w214:errorcluster)
          }
        }
      }
      frame #1 {
        n63 = flat-sequence {
          tunnel: w234 -> [w246]
          tunnel: w233 -> [w245]
          tunnel: w221 -> [w244]
          tunnel: w227 -> [w241]
          tunnel: [w243] -> w237
          tunnel: [w242] -> w236
          tunnel: [w241] -> w235
          tunnel: w220 -> [w240]
          tunnel: w219 -> [w239]
          tunnel: [w238] -> w218
          tunnel: [w282] -> w231
          tunnel: w237 -> [w284]
          tunnel: w236 -> [w283]
          tunnel: w235 -> [w281]
          tunnel: [w281] -> w226
          tunnel: [w280] -> w223
          tunnel: [w279] -> w217
          tunnel: w218 -> [w279]
          frame #0 {
            n64 = case shown="True" w241 {
              tunnel: w246 -> [w254 w273]
              tunnel: w245 -> [w252 w272]
              tunnel: [w251 w265] -> w242
              tunnel: w244 -> [_ _]
              tunnel: [w248 w264] -> w243
              tunnel: w240 -> [_ w259]
              tunnel: w239 -> [w247 w258]
              tunnel: [w247 w257] -> w238
              frame False {
                n65 = xnode "Invoke Method"("FPGA VI Reference In"=w254, "error in"=w252, "Number of Elements"=u32 0) -> ("FPGA VI Reference Out"=w250:refnum<k20>, "error out"=w249:errorcluster, "Elements Remaining"=w253:u32)  [unwired: 1 in, 1 out]
                n66 = xnode "Invoke Method"("FPGA VI Reference In"=w250, "error in"=w249, "Number of Elements"=w253) -> ("FPGA VI Reference Out"=w248:refnum<k20>, "error out"=w251:errorcluster)  [unwired: 1 in, 2 out]
              }
              frame True {
                n67 = xnode "Invoke Method"("FPGA VI Reference In"=w273, "error in"=w272, "Number of Elements"=u32 1024, "Timeout (ms)"=-1) -> ("FPGA VI Reference Out"=w267:refnum<k20>, "error out"=w266:errorcluster, "Data"=w269:fxp<+/-,12,12>[])  [unwired: 1 out]
                n68 = To Double Precision Float(number=w269) -> (double precision float=w260:dbl[])
                n69 = case shown="True" "Acrive Linearization" {
                  tunnel: w260 -> [_ w278]
                  tunnel: w259 -> [_ w277]
                  tunnel: w258 -> [w274 w276]
                  tunnel: [w274 w275] -> w257
                  frame False {
                  }
                  frame True {
                    n70 = RT FIFO Write(0:w277, 1:w278, 3:w276) -> (11:w275:errorcluster)  [unwired: 2 in, 3 out]
                  }
                }
                n71 = Split 1D Array(array=w260, index=512) -> (first subarray=→"First Signal (points) - Falling Triangular":dbl[], second subarray=→"Second Signal (points) - Rising Triangular":dbl[])
                n72 = xnode "Invoke Method"("FPGA VI Reference In"=w267, "error in"=w266, "Number of Elements"=u32 0) -> ("FPGA VI Reference Out"=w264:refnum<k20>, "error out"=w265:errorcluster)  [unwired: 1 in, 2 out]
              }
            }
          }
          frame #1 {
            n73 = case shown="True" w281 {
              tunnel: [w286 w289] -> w282
              tunnel: w284 -> [w285 w290]
              tunnel: w283 -> [w286 w288]
              tunnel: [w285 w287] -> w280
              frame False {
              }
              frame True {
                n74 = xnode "Read/Write Control"("FPGA VI Reference In"=w290, "error in"=w288, "snapshot"=FALSE) -> ("FPGA VI Reference Out"=w287:refnum<k20>, "error out"=w289:errorcluster)
              }
            }
          }
        }
        n75 = case shown="True" w230 {
          tunnel: w228 -> [w297 w318]
          tunnel: w229 -> [w294 w319]
          tunnel: [w293 w317] -> w232
          tunnel: w225 -> [_ w304]
          tunnel: w224 -> [_ w305]
          tunnel: w222 -> [_ w301]
          tunnel: w221 -> [_ w299]
          frame False {
            n76 = xnode "Invoke Method"("FPGA VI Reference In"=w297, "error in"=w294, "Number of Elements"=u32 0) -> ("FPGA VI Reference Out"=w295:refnum<k20>, "error out"=w292:errorcluster, "Elements Remaining"=w296:u32)  [unwired: 1 in, 1 out]
            n77 = xnode "Invoke Method"("FPGA VI Reference In"=w295, "error in"=w292, "Number of Elements"=w296) -> ("error out"=w293:errorcluster)  [unwired: 1 in, 3 out]
          }
          frame True {
            n78 = xnode "Invoke Method"("FPGA VI Reference In"=w318, "error in"=w319, "Number of Elements"=u32 512, "Timeout (ms)"=-1) -> ("FPGA VI Reference Out"=w315:refnum<k20>, "error out"=w316:errorcluster, "Data"=w321:fxp<+,44,44>[])  [unwired: 1 out]
            n79 = To Double Precision Float(number=w321) -> (double precision float=w320:dbl[])
            n80 = Square Root(x=w320) -> (sqrt(x)=w313:dbl[])
            n81 = Split 1D Array(array=w313, index=256) -> (first subarray=w311:dbl[], second subarray=w310:dbl[])
            "First FFT (bin)" <- w311
            "Second FFT (bin)" <- w310
            n82 = xnode "Invoke Method"("FPGA VI Reference In"=w315, "error in"=w316, "Number of Elements"=u32 0) -> ("error out"=w317:errorcluster)  [unwired: 1 in, 3 out]
            n83 = call "Distance-Velocity Calculation RT.vi"("First FFT"=w311, "Second FFT"=w310, "Windowing"=w301, "first FFT bin"=w304, "Sample Rate (S/s)"=w299, "last FFT bin"=w305) -> ("F_rise"=→"f_rise":dbl, "maxbin_firstFFT"=→"maxbin_firstFFT":i32, "maxbin_secondFFT"=→"maxbin_secondFFT":i32, "Distance (m)"=→"Distance (m)":dbl, "f_mean"=→"f_mean":dbl, "F_fall"=→"f_fall":dbl, "Velocity (m/s)"=→"Velocity (m/s)":dbl)  [unwired: 7 in]
          }
        }
      }
      frame #2 {
        n84 = case shown="True" w328 {
          tunnel: w325 -> [w331 w335]
          tunnel: [w331 w336] -> w324
          frame False {
          }
          frame True {
            n85 = Decrement(x="tieni premuto per") -> (x-1=w332:i32)
            n86 = Greater Or Equal?(x=w335, y=w332) -> (x >= y?=w334:bool)
            n87 = case shown="True" w334 {
              tunnel: w335 -> [w337 _]
              tunnel: [w338 0] -> w336
              frame False {
                n88 = Increment(x=w337) -> (x+1=w338:i32)
              }
              frame True {
                n89 = local write "Snapshot"(FALSE ("Snapshot")) -> ()
              }
            }
          }
        }
      }
    }
    n90 = node-c288() -> ()  [unwired: 1 in, 1 out]
  }
  n91 = node-c288(w50) -> ()  [unwired: 1 out]
  n92 = RT FIFO Delete(0:w30, 3:w29) -> (11:w28:errorcluster)  [unwired: 1 in]
  n93 = Merge Errors(w47, w48, w33, w28) -> (w31:errorcluster)
  n94 = flat-sequence {
    tunnel: w31 -> [w344]
    tunnel: w42 -> [w341]
    frame #0 {
      n95 = property class="Bool (strict)"(error in=w344, "Value"=FALSE ("stop")) -> (error out=w343:errorcluster)  [unwired: 1 in, 1 out]
      n96 = xnode "Invoke Method"("FPGA VI Reference In"=w341, "error in"=w343) -> ("FPGA VI Reference Out"=w346:refnum<k20>, "error out"=w345:errorcluster)
      n97 = xnode "Invoke Method"("FPGA VI Reference In"=w346, "error in"=w345) -> ("FPGA VI Reference Out"=w347:refnum<k20>, "error out"=w348:errorcluster)
      n98 = xnode "Close FPGA VI Reference"("FPGA VI Reference In"=w347, "error in"=w348) -> ()  [unwired: 1 out]
    }
  }
